vi "S2DS_ConditionForWriteToBuffer.vi"(3 "Measurement":bool, 6 "Scan parameters in":T1 {"Y data taking" items=["in both direction", "in up direction only", "in down direction only"]; "X data taking" items=["in both direction", "in up direction only", "in down direction only"]}) -> (1 "Update on?":bool, 2 "Measurement on?":bool)   [LabVIEW 2016]
uses:
  TYPE DEFS/S2DS_Sweep Info.ctl
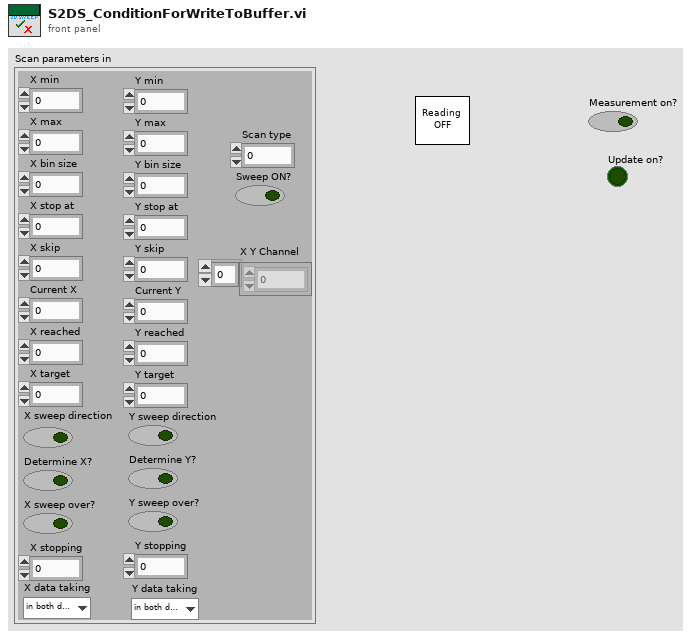
[diagram p1: front panel]
types:
  T1 = typedef "S2DS_Sweep Info.ctl" = cluster{"X min":ext, "X max":dbl, "Y min":dbl, "Y max":dbl, "X bin size":dbl, "Y bin size":dbl, "X stop at":dbl, "Y stop at":dbl, "X skip":u64, "Y skip":u64, "Current X":dbl, "Current Y":dbl, "X reached":i32, "Y reached":i32, "X target":dbl, "Y target":dbl, "Sweep ON?":bool, "X sweep direction":bool, "Y sweep direction":bool, "Determine X?":bool, "Determine Y?":bool, "X sweep over?":bool, "Y sweep over?":bool, "Scan type":i32, "X stopping":i32, "Y stopping":i32, "X Y Channel":u16[], "X data taking":u16, "Y data taking":u16}
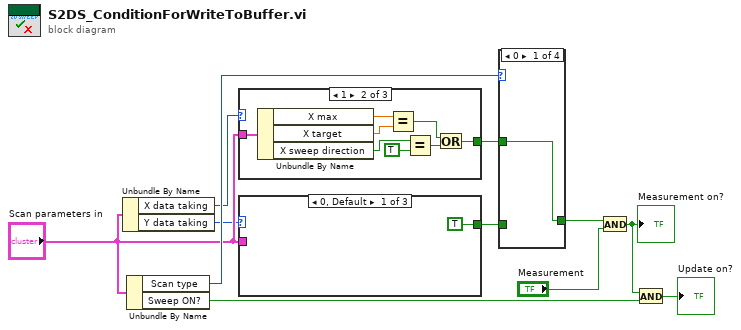
[diagram p0: block diagram]
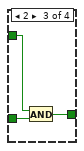
[diagram p3: hidden frame]
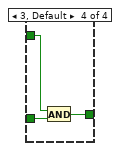
[diagram p4: hidden frame]
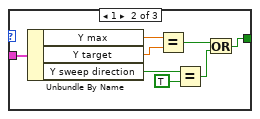
[diagram p5: hidden frame]
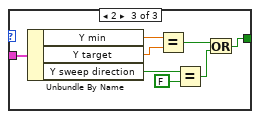
[diagram p6: hidden frame]
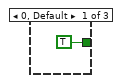
[diagram p7: hidden frame]
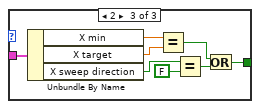
[diagram p8: hidden frame]
diagram:
  n1 = Unbundle By Name("Scan parameters in") -> ("X data taking"=w2:u16, "Y data taking"=w1:u16)
  n2 = Unbundle By Name("Scan parameters in") -> ("Scan type"=w9:i32, "Sweep ON?"=w6:bool)
  n3 = case shown="1" w2 {
    tunnel: [TRUE w13 w21] -> w10
    tunnel: "Scan parameters in" -> [_ w16 w24]
    frame 0, Default {
    }
    frame 1 {
      n4 = Unbundle By Name(w16) -> ("X max"=w20:dbl, "X target"=w19:dbl, "X sweep direction"=w18:bool)
      n5 = Equal?(x=w20, y=w19) -> (x = y?=w15:bool)
      n6 = Equal?(x=w18, y=TRUE) -> (x = y?=w14:bool)
      n7 = Or(x=w15, y=w14) -> (x .or. y?=w13:bool)
    }
    frame 2 {
      n8 = Unbundle By Name(w24) -> ("X min"=w28:ext, "X target"=w27:dbl, "X sweep direction"=w26:bool)
      n9 = Equal?(x=w28, y=w27) -> (x = y?=w23:bool)
      n10 = Equal?(x=w26, y=FALSE) -> (x = y?=w22:bool)
      n11 = Or(x=w23, y=w22) -> (x .or. y?=w21:bool)
    }
  }
  n12 = case shown="0, Default" w1 {
    tunnel: "Scan parameters in" -> [_ w37 w45]
    tunnel: [TRUE w30 w38] -> w11
    frame 0, Default {
    }
    frame 1 {
      n13 = Unbundle By Name(w37) -> ("Y max"=w36:dbl, "Y target"=w35:dbl, "Y sweep direction"=w34:bool)
      n14 = Equal?(x=w36, y=w35) -> (x = y?=w32:bool)
      n15 = Equal?(x=w34, y=TRUE) -> (x = y?=w31:bool)
      n16 = Or(x=w32, y=w31) -> (x .or. y?=w30:bool)
    }
    frame 2 {
      n17 = Unbundle By Name(w45) -> ("Y min"=w44:dbl, "Y target"=w43:dbl, "Y sweep direction"=w42:bool)
      n18 = Equal?(x=w44, y=w43) -> (x = y?=w40:bool)
      n19 = Equal?(x=w42, y=FALSE) -> (x = y?=w39:bool)
      n20 = Or(x=w40, y=w39) -> (x .or. y?=w38:bool)
    }
  }
  n21 = case shown="0" w9 {
    tunnel: [w46 w47 w48 w51] -> w7
    tunnel: w10 -> [w46 _ w50 w53]
    tunnel: w11 -> [_ w47 w49 w52]
    frame 0 {
    }
    frame 1 {
    }
    frame 2 {
      n22 = And(x=w50, y=w49) -> (x .and. y?=w48:bool)
    }
    frame 3, Default {
      n23 = And(x=w53, y=w52) -> (x .and. y?=w51:bool)
    }
  }
  n24 = And(x=w7, y="Measurement") -> (x .and. y?=w5:bool)
  "Measurement on?" <- w5
  n25 = And(x=w5, y=w6) -> (x .and. y?=→"Update on?":bool)
